vi "GV PreframegateScanGalvo.vi"() -> ()   [LabVIEW 2017]
panel:
  out "PreframegateScanGalvo":bool
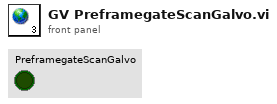
[diagram p1: front panel]
diagram:
